vi "toml_load_string.vi"() -> ()   [LabVIEW 2017]
panel:
  out "offset past match":i32
  out "before substring":string
  out "after substring":string
  out "match substring":string
  in  "offset (0)":i32
  in  "string":string
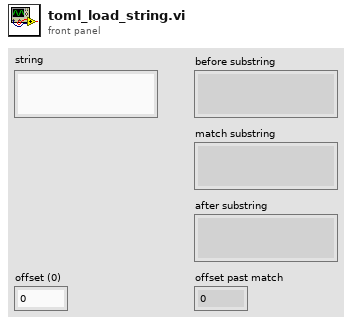
[diagram p1: front panel]
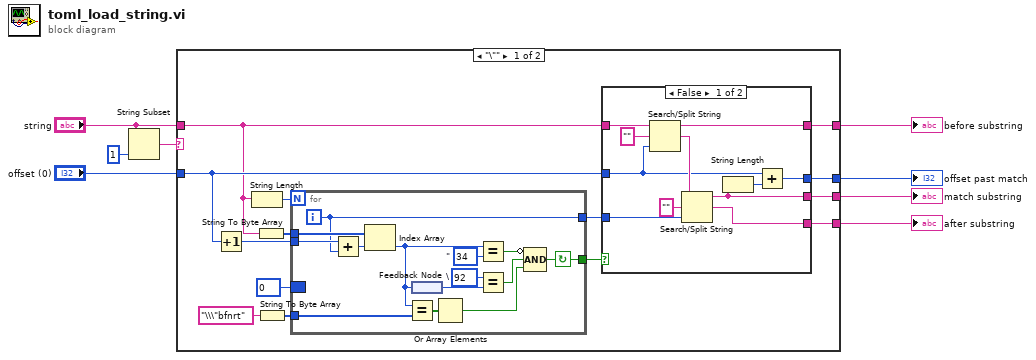
[diagram p0: block diagram]
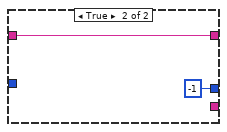
[diagram p2: hidden frame]
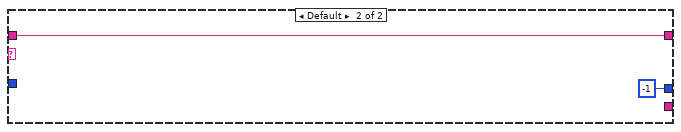
[diagram p3: hidden frame]
diagram:
  n1 = String Subset(string="string", length (rest)=1 ("length (rest)")) -> (substring=w2:string)  [unwired: 1 in]
  n2 = case shown="\"\\\"\"" w2 {
    tunnel: [w18 _] -> w8
    tunnel: [w17 _] -> w7
    tunnel: [w14 w51] -> w6
    tunnel: "offset (0)" -> [w13 _]
    tunnel: [w12 -1] -> w4
    tunnel: "string" -> [w10 w51]
    frame "\"" {
      n3 = Increment(x=w13) -> (x+1=w9:i32)
      n4 = String Length(string=w10) -> (length=w11:i32)
      n5 = String To Byte Array(string=w10) -> (unsigned byte array=w22:u8[])
      n6 = String To Byte Array(string="\\\"bfnrt") -> (unsigned byte array=w20:u8[])
      n7 = for {
        N: w11 -> [_]
        tunnel: w22 -> [w44]
        tunnel: w20 -> [w49]
        border: u8 0 -> [_]
        tunnel: [w40] -> w15
        tunnel: [w38] -> w16
        tunnel: w9 -> [w39]
        i -> [w38]
        stop <- w40 continue-if-true
        w45 = u8 34  # "
        w48 = u8 92  # \
        n8 = Add(x=w39, y=w38) -> (x+y=w36:i32)
        n9 = Index Array(array=w44, index=w36) -> (element=w37:u8)
        n10 = Equal?(x=w37, y=w49) -> (x = y?=w47:bool[])
        n11 = feedback #1() -> (w43:u8)
        n12 = feedback-in #1(w37) -> ()
        n13 = Or Array Elements(Boolean array=w47) -> (logical OR=w46:bool)
        n14 = Equal?(x=w37, y=w45) -> (x = y?=w41:bool)
        n15 = Equal?(x=w48, y=w43) -> (x = y?=w42:bool)
        n16 = Compound Arithmetic op=AND(invert w41, w42, w46) -> (w40:bool)
      }
      n17 = case shown="False" w15 {
        tunnel: [w26 _] -> w18
        tunnel: [w32 _] -> w17
        tunnel: w16 -> [w31 _]
        tunnel: w10 -> [w29 w35]
        tunnel: [w28 w35] -> w14
        tunnel: w13 -> [w24 _]
        tunnel: [w23 -1] -> w12
        frame False {
          n18 = Search/Split String(string=w29, search string/char (-)="", offset (0)=w24) -> (substring before match=w28:string, match + rest of string=w27:string)  [unwired: 1 out]
          n19 = Search/Split String(string=w27, search string/char (-)="", offset (0)=w31) -> (substring before match=w26:string, match + rest of string=w32:string)  [unwired: 1 out]
          n20 = String Length(string=w26) -> (length=w25:i32)
          n21 = Add(x=w24, y=w25) -> (x+y=w23:i32)
        }
        frame True {
        }
      }
    }
    frame Default {
    }
  }
  "match substring" <- w8
  "after substring" <- w7
  "before substring" <- w6
  "offset past match" <- w4
